vi "Write ZStateVCH.vi"(7 "OPC UA AI list":string[](array[string]), 8 "error in (no error)":errorcluster, 10 "Z_State":T1, 11 "OPC UA server refnum in":T5) -> (0 "error out":errorcluster, 3 "OPC UA server refnum out":T5)   [LabVIEW 2019, in "OPC addons.lvlib"]
uses:
  OPC addons.lvlib
  <vilib>/OPCUA/controls/OPC UA Server Refnum.ctl
  valves/ctl/Zs.ctl
  Heating/ctl/Y_source.ctl
  valves/ctl/Z_State_VCH.ctl
  valves/ctl/ZM_State_VCH.ctl
  valves/ctl/Z_short.ctl
  <vilib>/OPCUA/controls/Write Status.ctl
  <vilib>/OPCUA/server/Write Variant.vi
  <vilib>/OPCUA/NI OPC UA Server.lvlib
  valves/Valves.lvlib
  Heating/Heating.lvlib
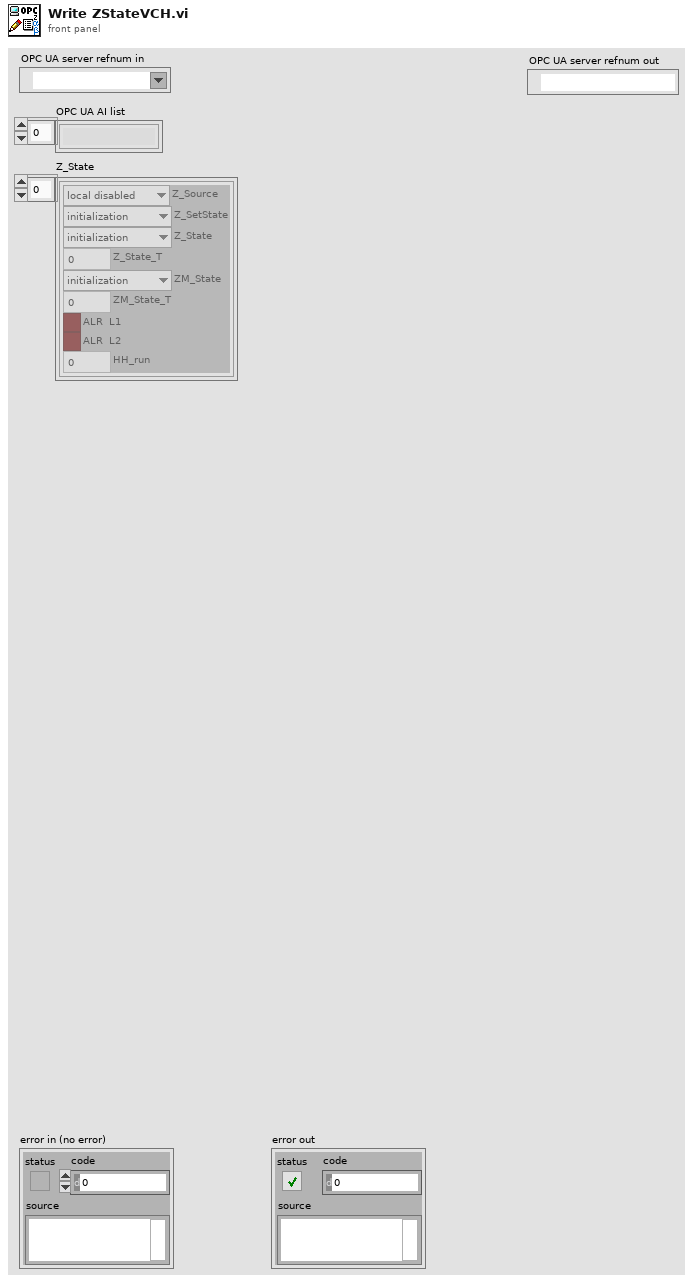
[diagram p1: front panel]
types:
  T1 = typedef "Valves.lvlib/Zs.ctl" = cluster{"Z_Source":T2, "Z_SetState":T3, "Z_State":T3, "Z_State_T":u32, "ZM_State":T4, "ZM_State_T":u32, "ALR  L1":bool, "ALR  L2":bool, "HH_run":i32}[]
  T2 = typedef "Heating.lvlib/Y_source.ctl" = enum8{"initialize", "local disabled", "local hand", "hand", "auto", "dist"}
  T3 = typedef "Valves.lvlib/Z_State_VCH.ctl" = enum8{"initialization", "alarm", "disabled", "not ready", "closed ready", "reserv", "reserv1", "reserv2", "reserv3", "check", "on min", "open", "on (closed)"}
  T4 = typedef "Valves.lvlib/ZM_State_VCH.ctl" = enum8{"initialization", "closed", "big_pause", "little_pause", "open", "close_cmd"}
  T5 = typedef "OPC UA Server Refnum.ctl" = refnum<k21>
  T6 = typedef "Valves.lvlib/Z_short.ctl" = cluster{"Z_Source":u8, "Z_SetState":u8, "Z_State":u8, "Z_State_T":u32, "ZM_State":u8, "ZM_State_T":u32, "ALR  L1":bool, "ALR  L2":bool, "HH_run":i32}
  T7 = typedef "Write Status.ctl" = u32
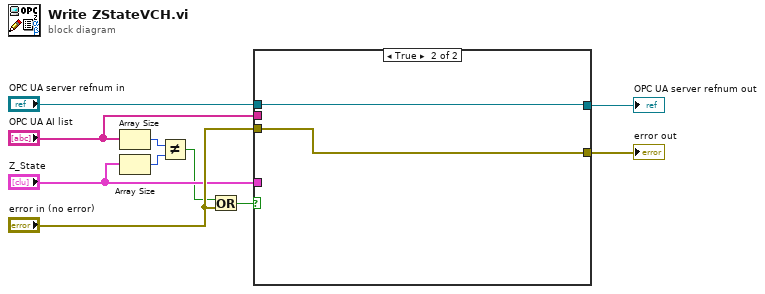
[diagram p0: block diagram]
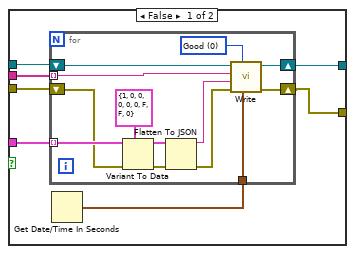
[diagram p2: hidden frame]
diagram:
  n1 = Array Size(array="OPC UA AI list") -> (size(s)=w5:i32)
  n2 = Array Size(array="Z_State") -> (size(s)=w4:i32)
  n3 = Not Equal?(x=w5, y=w4) -> (x != y?=w1:bool)
  n4 = Or(x=w1, y="error in (no error)") -> (x .or. y?=w6:bool)
  n5 = case shown="True" w6 {
    tunnel: "OPC UA server refnum in" -> [w14 w32]
    tunnel: [w16 w32] -> w9
    tunnel: [w15 w31] -> w8
    tunnel: "OPC UA AI list" -> [w13 _]
    tunnel: "error in (no error)" -> [w12 w31]
    tunnel: "Z_State" -> [w11 _]
    frame False {
      n6 = Get Date/Time In Seconds() -> (seconds since 1Jan1904=w17:timestamp)
      n7 = for {
        tunnel: w17 -> [w29]
        tunnel: w13 -> [w28] mode=indexing
        shift-right: [w26] -> w16
        shift-left: w14 -> [w30]
        shift-right: [w25] -> w15
        shift-left: w12 -> [w19]
        tunnel: w11 -> [w22] mode=indexing
        w24 = T7 0 items=["Good"=0, "Uncertain"=1073741824, "Uncertain_InitialValue"=1083310080, "Uncertain_LastUsableValue"=1083179008, "Uncertain_SensorNotAccurate"=1083375616, "Uncertain_EngineeringUnitsExceeded"=1083441152, "Bad"=2147483648, "Bad_NoCommunication"=2150694912, "Bad_NotReadable"=2151284736, "Bad_NotWritable"=2151350272, "Bad_OutOfRange"=2151415808, "Bad_WaitingForInitialData"=2150760448] ("node status")
        n8 = Variant To Data(error in=w19, type=T6 {"Z_Source"=1, "Z_SetState"=0, "Z_State"=0, "Z_State_T"=0, "ZM_State"=0, "ZM_State_T"=0, "ALR  L1"=FALSE, "ALR  L2"=FALSE, "HH_run"=0} ("Z"), Variant=w22) -> (data=w21:T6, error out=w20:errorcluster)
        n9 = Flatten To JSON(anything=w21, error in (no error)=w20) -> (JSON string=w27:string, 11:w23:errorcluster)  [unwired: 1 in]
        n10 = call-poly <vilib>:"Write.vi"("timestamp (current time)"=w29, "node status"=w24, "error in (no error)"=w23, "value"=w27, "node ID"=w28, "OPC UA server refnum in"=w30) -> ("error out"=w25:errorcluster, "OPC UA server refnum out"=w26:T5)  [unwired: 3 in, 1 out]
      }
    }
    frame True {
    }
  }
  "OPC UA server refnum out" <- w9
  "error out" <- w8
